vi "Actual Date and Time.vi"() -> (0 "Actual Time":string, 1 "Actual Date":string)   [LabVIEW 2019, in "EventsAbstract.lvclass"]
uses:
  EventsAbstract.lvclass
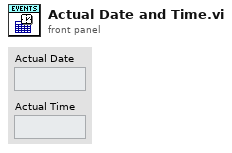
[diagram p1: front panel]
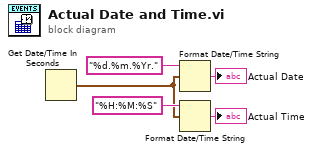
[diagram p0: block diagram]
diagram:
  n1 = Get Date/Time In Seconds() -> (seconds since 1Jan1904=w2:timestamp)
  n2 = Format Date/Time String(time format string (%c)="%d.%m.%Yr.", seconds (now)=w2) -> (date/time string=→"Actual Date":string)  [unwired: 1 in]
  n3 = Format Date/Time String(time format string (%c)="%H:%M:%S", seconds (now)=w2) -> (date/time string=→"Actual Time":string)  [unwired: 1 in]
